vi "Ch_data_title_pattern (SubVI).vi"(8 "error in":errorcluster, 9 "Единица измерений":string) -> (0 "error out":errorcluster, 2 "Path":path, 3 "Byte Stream File out":refnum<file>)   [LabVIEW 2015]
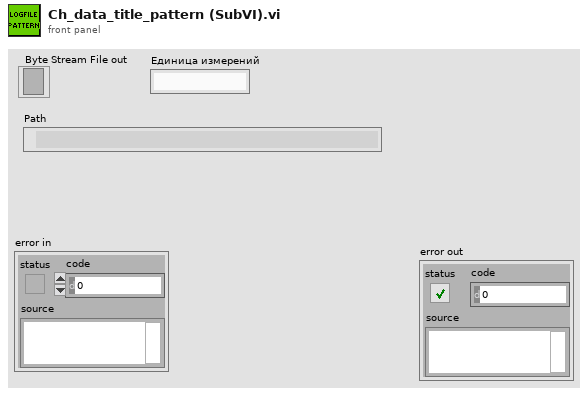
[diagram p1: front panel]
types:
  T1 = enum16{"open", "replace", "create", "open or create", "replace or create", "replace or create with confirmation"}
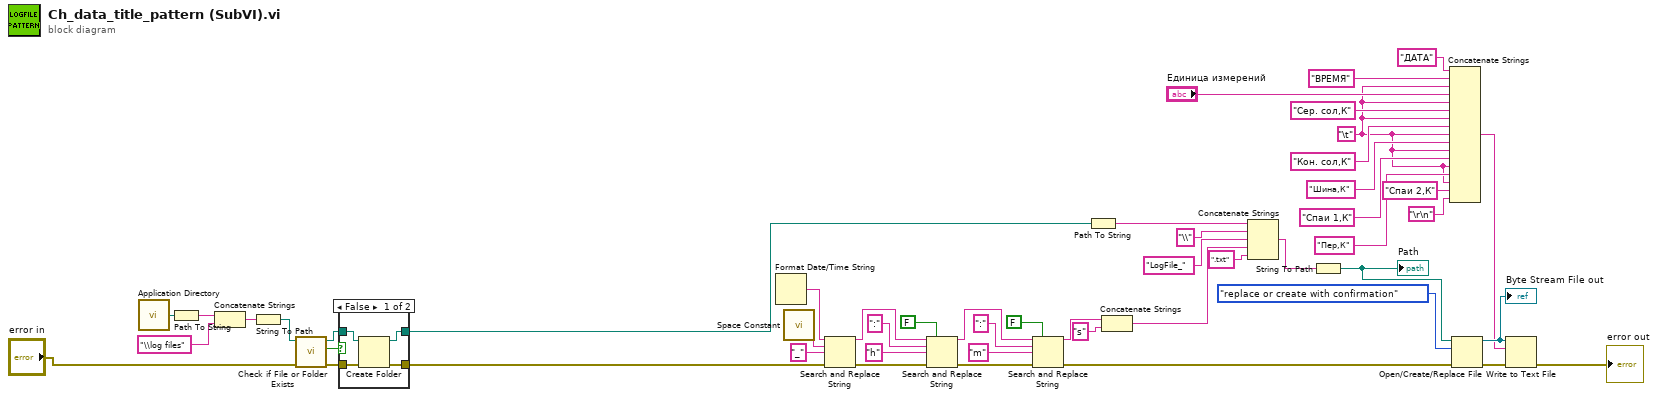
[diagram p0: block diagram]
diagram:
  w12 = "\t"
  n1 = call <vilib>:"Application Directory.vi"() -> ("Application Directory"=w5:path)
  n2 = Path To String(path=w5) -> (string=w4:string)
  n3 = Concatenate Strings(w4, "\\log files" ("replace string (\"\")")) -> (w2:string)
  n4 = String To Path(string=w2) -> (path=w1:path)
  n5 = call <vilib>:"Check if File or Folder Exists.vi"("error in (no error)"="error in", "path"=w1) -> ("error out"=w43:errorcluster, "file or folder exists?"=w42:bool, "dup path"=w44:path)  [unwired: 7 out]
  n6 = case shown="False" w42 {
    tunnel: [w54 w56] -> w6
    tunnel: w44 -> [w53 w56]
    tunnel: w43 -> [w52 w55]
    tunnel: [w51 w55] -> w7
    frame False {
      n7 = Create Folder(path (use dialog)=w53, error in=w52) -> (created path=w54:path, error out=w51:errorcluster)  [unwired: 2 out]
    }
    frame True {
    }
  }
  n8 = Format Date/Time String() -> (date/time string=w41:string)  [unwired: 3 out]
  n9 = call <vilib>:"Space Constant.vi"() -> ("String"=w22:string)
  n10 = Search and Replace String(input string=w41, search string=w22, replace string="_" ("replace string (\"\")"), error in=w7) -> (result string=w24:string, error out=w34:errorcluster)  [unwired: 6 out]
  n11 = Search and Replace String(replace all?=FALSE ("replace all? (F)"), input string=w24, search string=":", replace string="h" ("replace string (\"\")"), error in=w34) -> (result string=w31:string, error out=w35:errorcluster)  [unwired: 5 out]
  n12 = Search and Replace String(replace all?=FALSE ("replace all? (F)"), input string=w31, search string=":", replace string="m" ("replace string (\"\")"), error in=w35) -> (result string=w36:string, error out=w20:errorcluster)  [unwired: 5 out]
  n13 = Path To String(path=w6) -> (string=w32:string)
  n14 = Concatenate Strings(w36, "s" ("string")) -> (w39:string)
  n15 = Concatenate Strings(w32, "\\" ("string"), "LogFile_" ("string"), w39, ".txt" ("default name")) -> (w21:string)
  n16 = String To Path(string=w21) -> (path=w19:path)
  "Path" <- w19
  n17 = Concatenate Strings("ДАТА" ("string"), "ВРЕМЯ" ("string"), w12, "Единица измерений", w12, "Сер. сол,К" ("string"), w12, "Кон. сол,К" ("string"), w12, "Шина,К" ("string"), w12, "Спаи 1,К" ("string"), w12, "Пер,К" ("string"), w12, "Спаи 2,К" ("string"), "\r\n") -> (w46:string)
  n18 = Open/Create/Replace File(file path (use dialog)=w19, error in=w20, operation (0:open)=T1."replace or create with confirmation") -> (refnum out=w49:refnum<file>, error out=w47:errorcluster)  [unwired: 4 out]
  "Byte Stream File out" <- w49
  n19 = Write to Text File(file (use dialog)=w49, text=w46, error in=w47) -> (error out=→"error out":errorcluster)  [unwired: 3 out]
